vi "gen rand secenario.vi"(8 "error in (no error)":errorcluster, 10 "rand limits":T3={"# Number of emitters"=84, "# Number of frequency per emitter"={"Numeric"=0, "Numeric"=22}, "Frequency range"={"Numeric"=158778625.95419848, "Numeric"=2894656488.5496182}, "Frequency dispersion for each emitter"={"Numeric"=0.0, "Numeric"=1181732.2396298076}, "PRI range (Hz)"={"Numeric"=33.59056776941936, "Numeric"=576.0533087800792}, "Duty cycle - pulse in PRI"={"Numeric"=0.026717557251908396, "Numeric"=0.11832061068702289}, "Amplitude (dB)"={"Numeric"=-34.62595419847328, "Numeric"=-51.11450381679389}, "Modulation depth"={"Numeric"=19162.08437325717, "Numeric"=1181732.2396298076}, "CW"=TRUE, "LFM"=TRUE, "DOA (DEG)"={"Numeric"=0.0, "Numeric"=1181732.2396298076}, "start time (Sec)"=0.0, "end time (Sec)"=50.0, "BPSK"=TRUE, "QPSK"=TRUE} {"DOA (DEG)" scale=0.0..360.0 scale format="%#_6f"; "Modulation depth" scale=1000.0..10000000.0 scale format="%#_6pHz"; "Amplitude (dB)" scale format="%#_6fdB"; "Duty cycle - pulse in PRI" scale=0.0..1.0 scale format="%#_6f"; "PRI range (Hz)" scale=1.0..3000.0 scale format="%#_6pHz"; "Frequency dispersion for each emitter" scale=1000000.0..100000000.0 scale format="%#_6pHz"; "Frequency range" scale=975000000.0..2225000000.0 scale format="%#_4pHz"; "# Number of frequency per emitter" scale=0.01..3000.0; "# Number of emitters" scale=0.0..200.0}, 11 "device_type in":refnum<class "device_type.lvclass">) -> (0 "error out":errorcluster, 2 "transmitters":T1[](array[typedef]) {"t end" format="%#_3p"; "t start" format="%#_3p"; "DOA" format="%#_3p"; "mod depth" format="%#_3p"}, 3 "device_type out":refnum<class "device_type.lvclass">)   [LabVIEW 2021, in "device_type.lvclass"]
uses:
  device_type.lvclass
  pulse_tx_vis/random_limits.ctl
  pulse_tx_vis/emitter params.ctl
  pulse_tx_vis/mode_type.ctl
  device_type.lvclass/device_type.ctl
  <vilib>/numeric/Random Number (Range) DBL.vi
  <vilib>/numeric/Random Number (Range) U64.vi
  <vilib>/numeric/sub_Random U32.vi
panel:
  # "modulation \ntypes:"
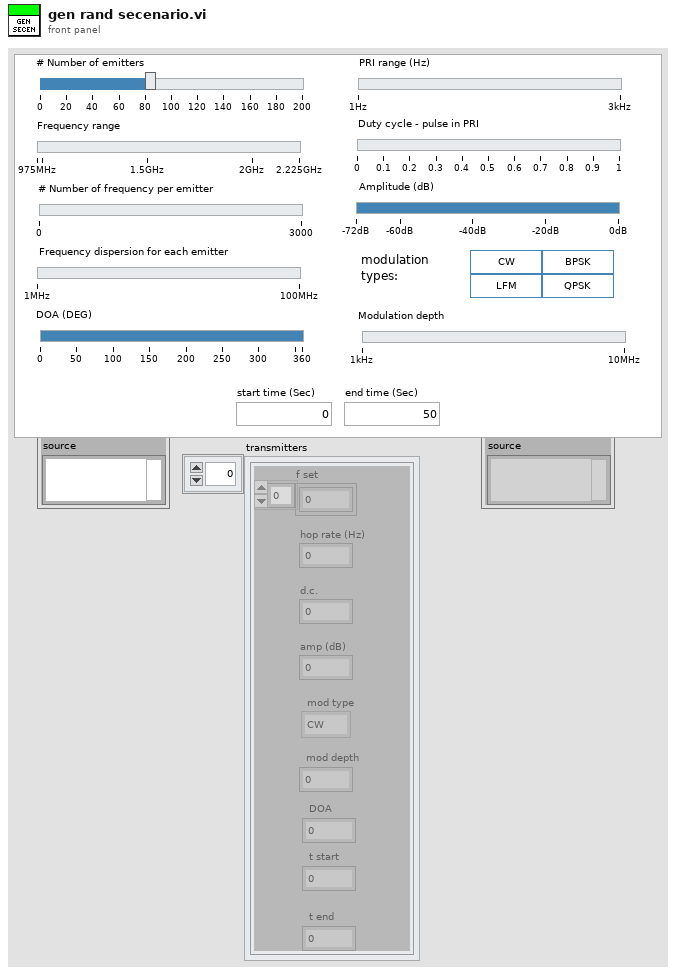
[diagram p1: front panel]
types:
  T1 = typedef "emitter params.ctl" = cluster{"f set":dbl[], "hop rate (Hz)":dbl, "d.c.":dbl, "amp (dB)":dbl, "mod type":T2, "mod depth":dbl, "DOA":dbl, "t start":dbl, "t end":dbl}
  T2 = typedef "mode_type.ctl" = enum8{"CW", "NC - CW", "NC - cw", "LFM", "BPSK", "QPSK"}
  T3 = typedef "random_limits.ctl" = cluster{"# Number of emitters":u32, "# Number of frequency per emitter":cluster{"Numeric":u32, "Numeric":u32}, "Frequency range":cluster{"Numeric":dbl, "Numeric":dbl}, "Frequency dispersion for each emitter":cluster{"Numeric":dbl, "Numeric":dbl}, "PRI range (Hz)":cluster{"Numeric":dbl, "Numeric":dbl}, "Duty cycle - pulse in PRI":cluster{"Numeric":dbl, "Numeric":dbl}, "Amplitude (dB)":cluster{"Numeric":dbl, "Numeric":dbl}, "Modulation depth":cluster{"Numeric":dbl, "Numeric":dbl}, "CW":bool, "LFM":bool, "DOA (DEG)":cluster{"Numeric":dbl, "Numeric":dbl}, "start time (Sec)":dbl, "end time (Sec)":dbl, "BPSK":bool, "QPSK":bool}
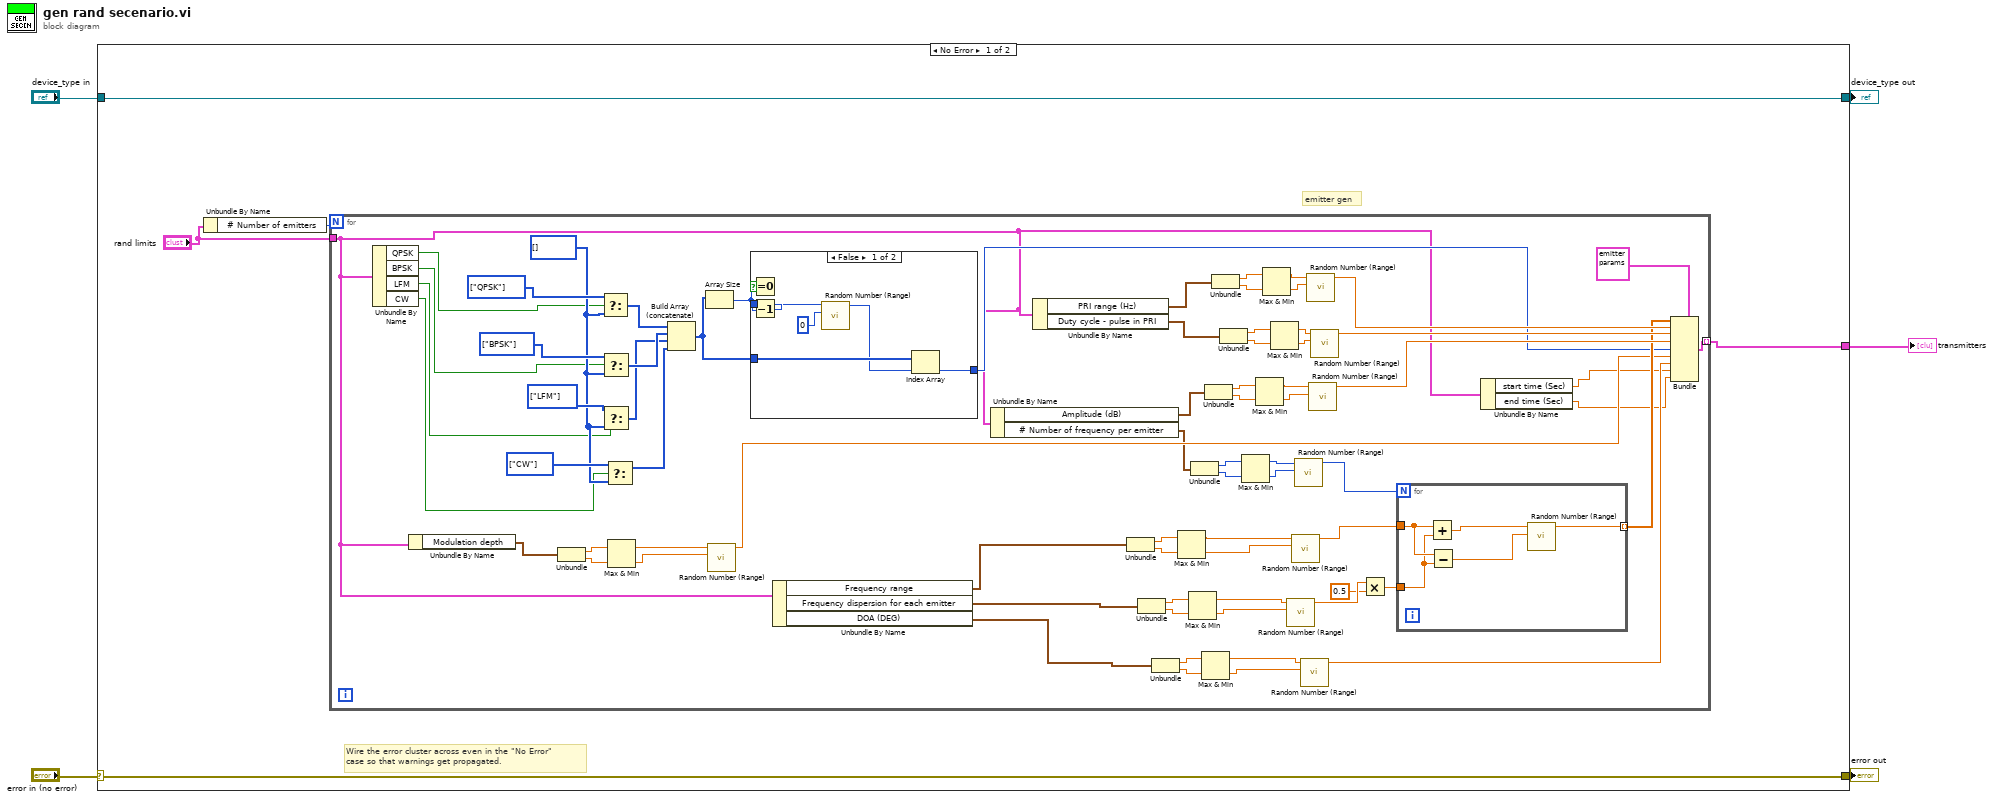
[diagram p0: block diagram]
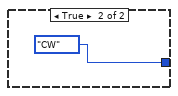
[diagram p2: hidden frame]
diagram:
  n1 = case shown="No Error" "error in (no error)" {
    selector: "error in (no error)" -> [w10 w97]
    tunnel: [w10 w97] -> w4
    tunnel: [w6 w96] -> w2
    tunnel: "device_type in" -> [w6 w96]
    tunnel: [w8 _] -> w1
    frame No Error {
      # "emitter gen"
      # "Wire the error cluster across even in the \"No Error\"\ncase so that warnings get propagated."
      n2 = Unbundle By Name("rand limits") -> ("# Number of emitters"=w9:u32)
      n3 = for {
        N: w9 -> [_]
        tunnel: [w75] -> w8 mode=indexing
        tunnel: "rand limits" -> [w13]
        w35 = T2[] [enum."QPSK"] items=["CW", "NC - CW", "NC - cw", "LFM", "BPSK", "QPSK"]
        w31 = T2[] [] items=["CW", "NC - CW", "NC - cw", "LFM", "BPSK", "QPSK"]
        w34 = T2[] [enum."BPSK"] items=["CW", "NC - CW", "NC - cw", "LFM", "BPSK", "QPSK"]
        w33 = T2[] [enum."LFM"] items=["CW", "NC - CW", "NC - cw", "LFM", "BPSK", "QPSK"]
        w32 = T2[] [enum."CW"] items=["CW", "NC - CW", "NC - cw", "LFM", "BPSK", "QPSK"]
        n4 = Unbundle By Name(w13) -> ("QPSK"=w25:bool, "BPSK"=w24:bool, "LFM"=w23:bool, "CW"=w22:bool)
        n5 = Unbundle By Name(w13) -> ("Modulation depth"=w12:cluster{"Numeric":dbl, "Numeric":dbl})
        n6 = Unbundle(w12) -> ("Numeric"=w49:dbl, "Numeric"=w48:dbl)
        n7 = Select(t=w35, s=w25, f=w31) -> (s? t:f=w45:T2[])
        n8 = Select(t=w34, s=w24, f=w31) -> (s? t:f=w44:T2[])
        n9 = Select(t=w33, s=w23, f=w31) -> (s? t:f=w43:T2[])
        n10 = Select(t=w32, s=w22, f=w31) -> (s? t:f=w42:T2[])
        n11 = Max & Min(x=w49, y=w48) -> (max(x,y)=w47:dbl, min(x,y)=w46:dbl)
        n12 = Build Array (concatenate)(w45, w44, w43, w42) -> (w41:T2[])
        n13 = Array Size(array=w41) -> (size(s)=w37:i32)
        n14 = call-poly <vilib>:"Random Number (Range).vi"("lower bound (0)"=w46, "upper bound (100)"=w47) -> ("number"=w38:dbl)  [unwired: 9 in]
        n15 = Equal To 0?(x=w37) -> (x = 0?=w39:bool)
        n16 = Decrement(x=w37) -> (x-1=w36:i32)
        n17 = case shown="False" w39 {
          tunnel: w41 -> [w88 _]
          tunnel: [w86 mode_type."CW" ("mod type")] -> w40
          tunnel: w36 -> [w85 _]
          frame False {
            n18 = call-poly <vilib>:"Random Number (Range).vi"("lower bound (0)"=u64 0, "upper bound (100)"=w85) -> ("number"=w87:u64)  [unwired: 9 in]
            n19 = Index Array(array=w88, index=w87) -> (element=w86:T2)
          }
          frame True {
          }
        }
        n20 = Unbundle By Name(w13) -> ("Frequency range"=w11:cluster{"Numeric":dbl, "Numeric":dbl}, "Frequency dispersion for each emitter"=w16:cluster{"Numeric":dbl, "Numeric":dbl}, "DOA (DEG)"=w17:cluster{"Numeric":dbl, "Numeric":dbl})
        n21 = Unbundle By Name(w13) -> ("Amplitude (dB)"=w19:cluster{"Numeric":dbl, "Numeric":dbl}, "# Number of frequency per emitter"=w18:cluster{"Numeric":u32, "Numeric":u32})
        n22 = Unbundle By Name(w13) -> ("PRI range (Hz)"=w21:cluster{"Numeric":dbl, "Numeric":dbl}, "Duty cycle - pulse in PRI"=w20:cluster{"Numeric":dbl, "Numeric":dbl})
        n23 = Unbundle(w11) -> ("Numeric"=w57:dbl, "Numeric"=w56:dbl)
        n24 = Unbundle(w16) -> ("Numeric"=w52:dbl, "Numeric"=w53:dbl)
        n25 = Unbundle(w17) -> ("Numeric"=w28:dbl, "Numeric"=w27:dbl)
        n26 = Max & Min(x=w57, y=w56) -> (max(x,y)=w55:dbl, min(x,y)=w54:dbl)
        n27 = Max & Min(x=w52, y=w53) -> (max(x,y)=w51:dbl, min(x,y)=w50:dbl)
        n28 = Unbundle(w18) -> ("Numeric"=w60:u32, "Numeric"=w61:u32)
        n29 = Max & Min(x=w28, y=w27) -> (max(x,y)=w29:dbl, min(x,y)=w30:dbl)
        n30 = Unbundle(w19) -> ("Numeric"=w71:dbl, "Numeric"=w70:dbl)
        n31 = Unbundle(w21) -> ("Numeric"=w65:dbl, "Numeric"=w64:dbl)
        n32 = Unbundle(w20) -> ("Numeric"=w68:dbl, "Numeric"=w69:dbl)
        n33 = Max & Min(x=w60, y=w61) -> (max(x,y)=w59:u32, min(x,y)=w58:u32)
        n34 = Max & Min(x=w71, y=w70) -> (max(x,y)=w73:dbl, min(x,y)=w72:dbl)
        n35 = Max & Min(x=w65, y=w64) -> (max(x,y)=w63:dbl, min(x,y)=w62:dbl)
        n36 = Max & Min(x=w68, y=w69) -> (max(x,y)=w67:dbl, min(x,y)=w66:dbl)
        n37 = call-poly <vilib>:"Random Number (Range).vi"("lower bound (0)"=w50, "upper bound (100)"=w51) -> ("number"=w80:dbl)  [unwired: 9 in]
        n38 = call-poly <vilib>:"Random Number (Range).vi"("lower bound (0)"=w54, "upper bound (100)"=w55) -> ("number"=w78:dbl)  [unwired: 9 in]
        n39 = call-poly <vilib>:"Random Number (Range).vi"("lower bound (0)"=w58, "upper bound (100)"=w59) -> ("number"=w74:u64)  [unwired: 9 in]
        n40 = call-poly <vilib>:"Random Number (Range).vi"("lower bound (0)"=w30, "upper bound (100)"=w29) -> ("number"=w26:dbl)  [unwired: 9 in]
        n41 = call-poly <vilib>:"Random Number (Range).vi"("lower bound (0)"=w62, "upper bound (100)"=w63) -> ("number"=w83:dbl)  [unwired: 9 in]
        n42 = call-poly <vilib>:"Random Number (Range).vi"("lower bound (0)"=w72, "upper bound (100)"=w73) -> ("number"=w81:dbl)  [unwired: 9 in]
        n43 = call-poly <vilib>:"Random Number (Range).vi"("lower bound (0)"=w66, "upper bound (100)"=w67) -> ("number"=w82:dbl)  [unwired: 9 in]
        n44 = Multiply(x=w80, y=0.5) -> (x*y=w77:dbl)
        n45 = for {
          N: w74 -> [_]
          tunnel: w78 -> [w95]
          tunnel: w77 -> [w94]
          tunnel: [w91] -> w76 mode=indexing
          n46 = Add(x=w95, y=w94) -> (x+y=w92:dbl)
          n47 = Subtract(x=w95, y=w94) -> (x-y=w93:dbl)
          n48 = call-poly <vilib>:"Random Number (Range).vi"("lower bound (0)"=w93, "upper bound (100)"=w92) -> ("number"=w91:dbl)  [unwired: 9 in]
        }
        n49 = Unbundle By Name(w13) -> ("start time (Sec)"=w15:dbl, "end time (Sec)"=w14:dbl)
        n50 = Bundle(cluster=T1 {"f set"=[1000000.0], "hop rate (Hz)"=300000.0, "d.c."=0.0, "amp (dB)"=-20.0, "mod type"=enum."CW", "mod depth"=0.0, "DOA"=0.0, "t start"=0.0, "t end"=0.0} ("Cluster"), "f set"=w76, "hop rate (Hz)"=w83, "d.c."=w82, "amp (dB)"=w81, "mod type"=w40, "mod depth"=w38, "DOA"=w26, "t start"=w15, "t end"=w14) -> (w75:T1)
      }
    }
    frame Error {
    }
  }
  "error out" <- w4
  "device_type out" <- w2
  "transmitters" <- w1
